vi "PH_Beckhoff_StepMot.set Postion.vi"(0 "VI in":refnum<vi>, 1 "AMS Net ID":T1, 2 "Axis":i32, 3 "ADS Error in":i32, 4 "Wanted Position":i32, 5 "error in (no error)":errorcluster) -> (14 "VI out":refnum<vi>, 15 "AMS Net ID out":T1, 17 "ADS Error out":i32, 18 "ok?":bool, 19 "error out":errorcluster)   [LabVIEW 2014, in "PH_Beckhoff_StepMot.lvlib"]
uses:
  PH_Beckhoff_StepMot.lvlib
  instr.lib/Beckhoff/Helpers/Beckhoff Access.ctl
  instr.lib/Beckhoff/Read and Write Data/Step Motor Klemmen/Beckhoff.Step Motor - Control Word.ctl
  instr.lib/Beckhoff/Beckhoff - Driver np.lvlib
  PH_Basics/PH_Stepmotor_BaseClass/PH_Stepmotor_BaseClass.lvlib
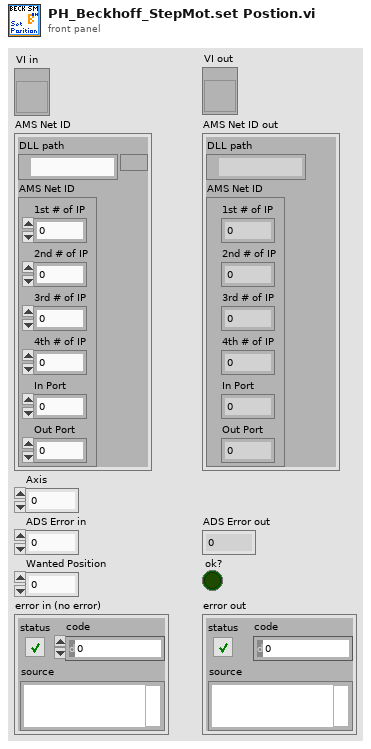
[diagram p1: front panel]
types:
  T1 = typedef "Beckhoff - Driver np.lvlib/Beckhoff Access.ctl" = cluster{"DLL path":path, "AMS Net ID":cluster{"1st # of IP":u8, "2nd # of IP":u8, "3rd # of IP":u8, "4th # of IP":u8, "In Port":u8, "Out Port":u8}}
  T2 = typedef "Beckhoff - Driver np.lvlib/Beckhoff.Step Motor - Control Word.ctl" = cluster{"en Latch C":bool, "en Latch Input 1":bool, "en Latch Input 2":bool, "en Latch Rise Edge":bool, "en Latch Fall Edge":bool, "Get Latch Data":bool, "Toggle Latch Data":bool, "Get Position Error":bool, "Get Encoder Position":bool, "Dis mixed Decay":bool, "Set Pos":bool, "Reduced Current":bool, "Reduced Current (drivng)":bool, "Clear Position":bool, "Set Position in Process Data":bool, "N/A":bool}
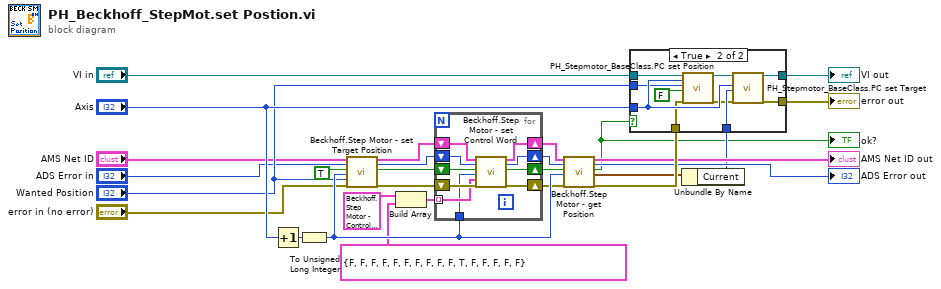
[diagram p0: block diagram]
diagram:
  n1 = Increment(x="Axis") -> (x+1=w26:i32)
  n2 = To Unsigned Long Integer(number=w26) -> (unsigned 32bit integer=w27:u32)
  n3 = call "Beckhoff.Step Motor - set Target Position.vi"("AMS Net ID in"="AMS Net ID", "ADS Error in (0)"="ADS Error in", "Write?"=TRUE, "# of Klemme [1, ...]"=w27, "Target Position"="Wanted Position", "error in (no error)"="error in (no error)") -> ("AMS Net ID out"=w2:T1, "ADS Error out"=w7:i32, "Write successful?"=w6:bool, "error out"=w8:errorcluster)  [unwired: 10 in]
  n4 = Build Array(T2 {"en Latch C"=FALSE, "en Latch Input 1"=FALSE, "en Latch Input 2"=FALSE, "en Latch Rise Edge"=FALSE, "en Latch Fall Edge"=FALSE, "Get Latch Data"=FALSE, "Toggle Latch Data"=FALSE, "Get Position Error"=FALSE, "Get Encoder Position"=FALSE, "Dis mixed Decay"=FALSE, "Set Pos"=FALSE, "Reduced Current"=FALSE, "Reduced Current (drivng)"=FALSE, "Clear Position"=FALSE, "Set Position in Process Data"=FALSE, "N/A"=FALSE} ("Control Word"), T2 {"en Latch C"=FALSE, "en Latch Input 1"=FALSE, "en Latch Input 2"=FALSE, "en Latch Rise Edge"=FALSE, "en Latch Fall Edge"=FALSE, "Get Latch Data"=FALSE, "Toggle Latch Data"=FALSE, "Get Position Error"=FALSE, "Get Encoder Position"=FALSE, "Dis mixed Decay"=FALSE, "Set Pos"=TRUE, "Reduced Current"=FALSE, "Reduced Current (drivng)"=FALSE, "Clear Position"=FALSE, "Set Position in Process Data"=FALSE, "N/A"=FALSE} ("Control Word")) -> (w4:T2[])
  n5 = for {
    tunnel: w4 -> [w32] mode=indexing
    shift-right: [w37] -> w23
    shift-left: w8 -> [w38]
    shift-right: [w33] -> w21
    shift-left: w7 -> [w35]
    tunnel: w27 -> [w31]
    shift-right: [w30] -> w19
    shift-left: w2 -> [w36]
    shift-right: [w29] -> w16
    shift-left: w6 -> [w34]
    n6 = call "Beckhoff.Step Motor - set Control Word.vi"("AMS Net ID in"=w36, "ADS Error in (0)"=w35, "Write?"=w34, "# of Klemme [1, ...]"=w31, "Control Word"=w32, "error in (no error)"=w38) -> ("AMS Net ID out"=w30:T1, "ADS Error out"=w33:i32, "Write successful?"=w29:bool, "error out"=w37:errorcluster)  [unwired: 10 in]
  }
  n7 = call "Beckhoff.Step Motor - get Position.vi"("AMS Net ID in"=w19, "ADS Error in (0)"=w21, "Read?"=w16, "# of Klemme [1, ...]"=w27, "error in (no error)"=w23) -> ("AMS Net ID out"=→"AMS Net ID out":T1, "ADS Error out"=→"ADS Error out":i32, "Read successful?"=w1:bool, "Position"=w17:cluster{"Target":i32, "Current":i32}, "error out"=w24:errorcluster)  [unwired: 10 in]
  "ok?" <- w1
  n8 = Unbundle By Name(w17) -> ("Current"=w18:i32)
  n9 = case shown="True" w1 {
    tunnel: "Axis" -> [_ w50]
    tunnel: w24 -> [w39 w49]
    tunnel: w18 -> [_ w48]
    tunnel: "VI in" -> [w40 w47]
    tunnel: [w39 w45] -> w13
    tunnel: [w40 w44] -> w12
    tunnel: "Wanted Position" -> [_ w42]
    frame False {
    }
    frame True {
      n10 = call "PH_Stepmotor_BaseClass.PC set Position.vi"("i ref in"=w47, "axis"=w50, "Position to set"=w42, "Set?"=FALSE, "error in (no error)"=w49) -> ("i ref out"=w43:refnum<vi>, "error out"=w46:errorcluster)  [unwired: 12 in, 1 out]
      n11 = call "PH_Stepmotor_BaseClass.PC set Target.vi"("VI in"=w43, "axis"=w50, "Targetposition to set"=w48, "error in (no error)"=w46) -> ("VI out"=w44:refnum<vi>, "error out"=w45:errorcluster)  [unwired: 14 in]
    }
  }
  "error out" <- w13
  "VI out" <- w12
